vi "unregisterPublisher.vi"(1 "Parameters":T2) -> (2 "Error out":errorcluster, 3 "Reply":T1, 4 "Reply":string, 5 "registerPublisher":string)   [LabVIEW 2013]
uses:
  _ROSDefinition.vi
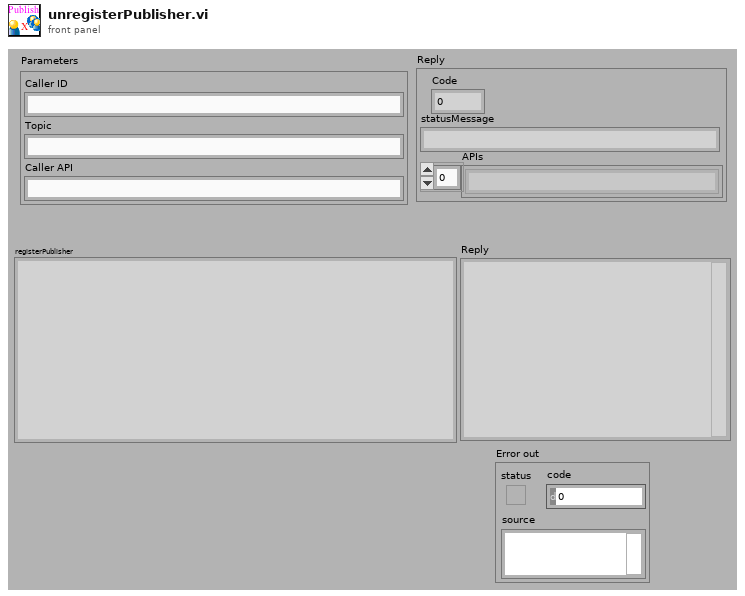
[diagram p1: front panel]
types:
  T1 = cluster{"Code":i8, "statusMessage":string, "APIs":string[]}
  T2 = cluster{"Caller ID":string, "Topic":string, "Caller API":string}
  T3 = cluster{"Code":i8, "statusMessage":string, "APIs":string[]}[]
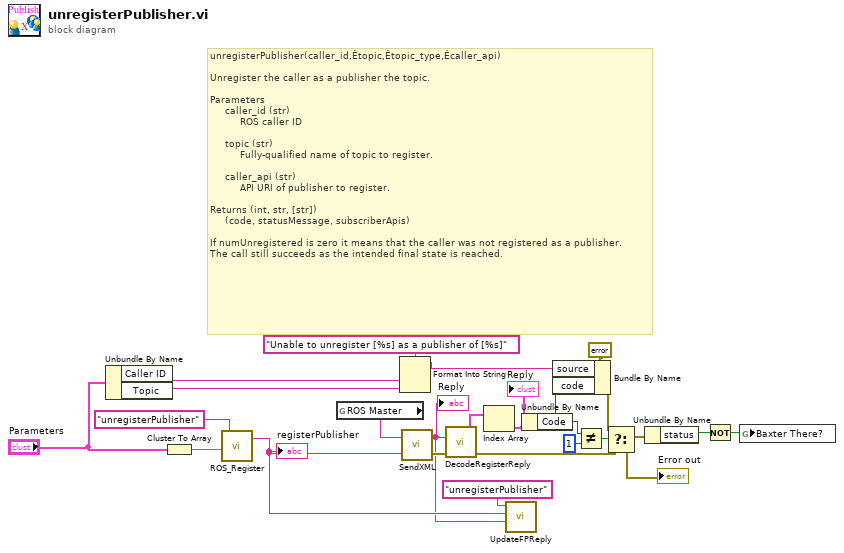
[diagram p0: block diagram]
diagram:
  # "unregisterPublisher(caller_id,Êtopic,Êtopic_type,Êcaller_api)\n\nUnregister the caller as a publisher the topic. \n\nParameters \n     caller_id (str) \n          ROS caller ID\n\n     topic (str) \n          Fully-qualified name of topic to register.\n\n     caller_api (str) \n          API URI of publisher to register.\n\nReturns (int, str, [str]) \n     (code, statusMessage, subscriberApis) \n\nIf numUnregistered is zero it means that the caller was not registered as a publisher. \nThe call still succeeds as the intended final state is reached."
  n1 = Unbundle By Name("Parameters") -> ("Caller ID"=w20:string, "Topic"=w19:string)
  n2 = Cluster To Array(cluster="Parameters") -> (array=w4:string[])
  n3 = call "ROS_Register.vi"("Parameters"=w4, "Method Name"="unregisterPublisher") -> ("registerSubscriber"=w2:string)  [unwired: 1 in]
  "registerPublisher" <- w2
  n4 = global read "_ROSDefinition.vi" "ROS Master"() -> (w23:string)
  n5 = Format Into String(format string="Unable to unregister [%s] as a publisher of [%s]" ("source"), w20, w19) -> (resulting string=w7:string)  [unwired: 2 in, 1 out]
  n6 = call "SendXML.vi"("Send"=w2, "URI in"=w23) -> ("error out"=w8:errorcluster, "Reply"=w1:string)
  "Reply" <- w1
  n7 = call "DecodeRegisterReply.vi"("error in (no error)"=w8, "Response"=w1) -> ("error out"=w12:errorcluster, "Reply"=w16:T3)
  n8 = Index Array(array=w16) -> (element=w15:T1)  [unwired: 1 in]
  "Reply" <- w15
  n9 = call "UpdateFPReply.vi"("Reply"=w1, "Sent"=w2, "method"="unregisterPublisher" ("name (unnamed)")) -> ()  [unwired: 3 in]
  n10 = Unbundle By Name(w15) -> ("Code"=w11:i8)
  n11 = Bundle By Name(cluster=errorcluster {"status"=TRUE, "code"=0, "source"=" Error"} ("t"), "source"=w7, "code"=w11) -> (w10:errorcluster)
  n12 = Not Equal?(x=w11, y=i8 1) -> (x != y?=w13:bool)
  n13 = Select(t=w10, s=w13, f=w12) -> (s? t:f=w9:errorcluster)
  "Error out" <- w9
  n14 = Unbundle By Name(w9) -> ("status"=w17:bool)
  n15 = Not(x=w17) -> (.not. x?=w18:bool)
  n16 = global write "_ROSDefinition.vi" "Baxter There?"(w18) -> ()
